vi "Control - Generic - Next Cycle CA50 Host.vi"() -> ()   [LabVIEW 2015, in "ECS-Host.lvlib"]
uses:
  ECS-Host.lvlib
  <vilib>/addons/Software Calibration Management/XControls/TBL2D.xctl
panel:
  out "ReadyAngle":sgl[](array[numeric]) caption="[DBTDC]"
  in  "MaxReadyAngle":sgl caption="[DBTDC]"
  out "CA50ControlOutputValid":u8
  out "_CA50 Control Output Valid":bool[](array[boolean]) caption="CA50ControlOutputValid"
  in  "CA50PIDTimeout":u32 caption="[ms]"
  out "CA50ControlOutput":sgl[](array[numeric]) caption="[CAD]"
  out "CA50":sgl[](array[numeric]) caption="[DATDC]"
  out "_Channel Labels":string[](array[string]) caption="[]"
  in  "FeedbackControlEnable":bool
  in  "CA50_Td":sgl caption="[min]"
  in  "CA50_Ti":sgl caption="[min]"
  in  "CA50_Kp":sgl caption="[CAD/CAD]"
  in  "CA50_PIDMin":sgl caption="[CAD]"
  in  "CA50_PIDMax":sgl caption="[CAD]"
  in  "CA50Stp_ManE":bool
  in  "CA50Stp_Man":sgl caption="[bar]"
  out "CA50Stp_Des":sgl caption="[bar]"
  in  "CA50Stp_Tbl":cluster{"X":sgl[], "Y":sgl[], "Z":sgl[][]}(xcontrol) caption="[]"
  # "Next-Cycle PID Tuning"
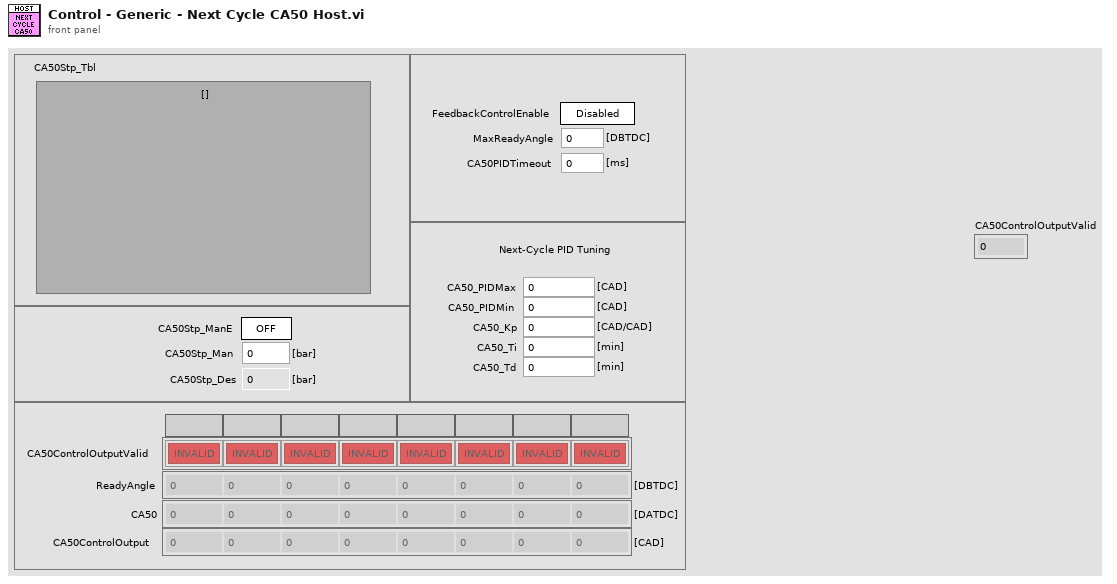
[diagram p1: front panel]
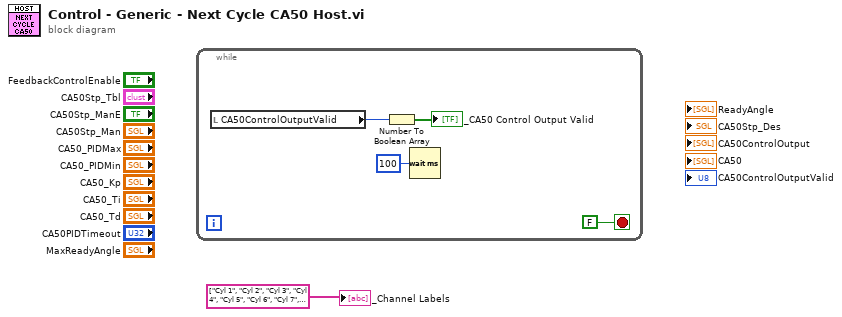
[diagram p0: block diagram]
diagram:
  n1 = while {
    stop <- FALSE stop-if-true
    n2 = local read "CA50ControlOutputValid"() -> (w2:u8)
    n3 = Number To Boolean Array(number=w2) -> (Boolean array=→"_CA50 Control Output Valid":bool[])
    n4 = Wait (ms)(milliseconds to wait=u32 100) -> ()  [unwired: 1 out]
  }
  "_Channel Labels" <- string[] ["Cyl 1", "Cyl 2", "Cyl 3", "Cyl 4", "Cyl 5", "Cyl 6", "Cyl 7", "Cyl 8"] ("_Pulse Gen Labels 2")
